vi "writeMsg.vi"(0 "ID":u32 format="%x", 1 "ID Type":enum16{"Standard", "Extended"}(ring), 2 "SPI Config In":T1, 3 "Data to Write":u8[](array[numeric])=[0, 0, 0, 0, 0, 0, 0, 0] format="%x", 4 "Frames to Write":u8) -> (5 "SPI Config Out":T1)   [LabVIEW 2019]
uses:
  SPI/SPI Config.ctl
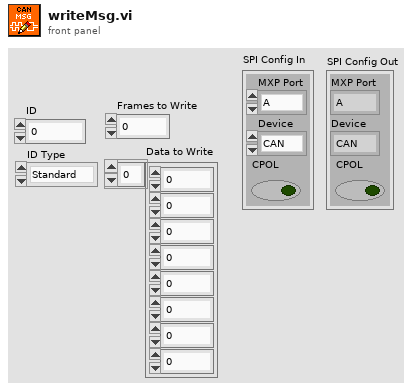
[diagram p1: front panel]
types:
  T1 = typedef "SPI Config.ctl" = cluster{"MXP Port":enum16{"A", "B"}, "Device":enum16{"CAN", "ENC", "IMU1", "IMU2"}, "CPOL":bool}
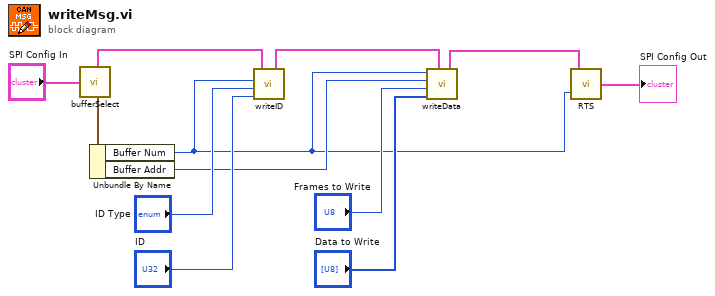
[diagram p0: block diagram]
diagram:
  n1 = call "bufferSelect.vi"("SPI Config In"="SPI Config In") -> ("SPI Config Out"=w11:T1, "Buffer"=w9:cluster{"Buffer Num":u8, "Buffer Addr":u8})
  n2 = Unbundle By Name(w9) -> ("Buffer Num"=w2:u8, "Buffer Addr"=w6:u8)
  n3 = call "writeID.vi"("ID"="ID", "ID Type"="ID Type", "Buffer Num"=w2, "SPI Config In"=w11) -> ("SPI Config Out"=w10:T1)
  n4 = call "writeData.vi"("Buffer Num"=w2, "Buffer Addr"=w6, "Frames to Write"="Frames to Write", "Data to Write"="Data to Write", "SPI Config In"=w10) -> ("SPI Config Out"=w3:T1)
  n5 = call "RTS.vi"("Reg. Select"=w2, "SPI Config In"=w3) -> ("SPI Config Out"=→"SPI Config Out":T1)
